vi "SS Current Test.vi"(6 "Lower Limit 2":dbl[](array[numeric])=[18.0, 18.0, 18.0, 18.0, 18.0, 18.0, 18.0, 18.0, 18.0, -1.0, -1.0, -1.0, -1.0, -1.0, -1.0, -1.0, -1.0, -1.0, 3.6, 3.6, 3.6, 3.6, 3.6, 3.6, -1.0, -1.0, -1.0, -1.0], 8 "Lower Limit":dbl[](array[numeric])=[18.0, 18.0, 18.0, 18.0, 18.0, 18.0, 18.0, 18.0, 18.0, -1.0, -1.0, -1.0, -1.0, -1.0, -1.0, -1.0, -1.0, -1.0, 3.6, 3.6, 3.6, 3.6, 3.6, 3.6, -1.0, -1.0, -1.0, -1.0], 9 "Y 2":dbl[](array[numeric]), 10 "Y":dbl[](array[numeric]), 11 "Upper Limit":dbl[](array[numeric])=[50.0, 50.0, 27.0, 27.0, 27.0, 27.0, 27.0, 27.0, 27.0, 27.0, 27.0, 1.0, 1.0, 1.0, 1.0, 1.0, 4.4, 4.4, 4.4, 4.4, 4.4, 4.4, 4.4, 4.4, 4.4, 4.4, 1.0, 1.0]) -> (2 "Out of Bounds":bool, 3 "Waveform Chart":waveform(dbl)[](graph))   [LabVIEW 2012]
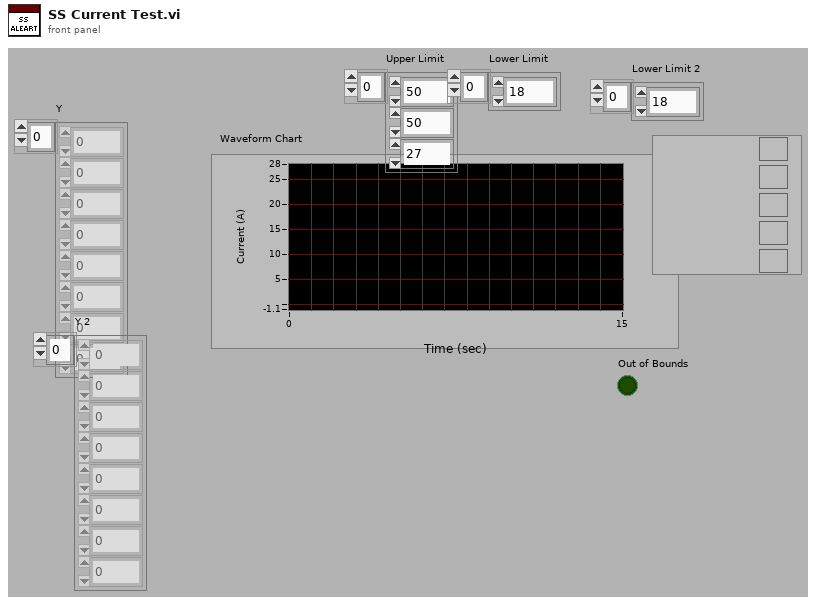
[diagram p1: front panel]
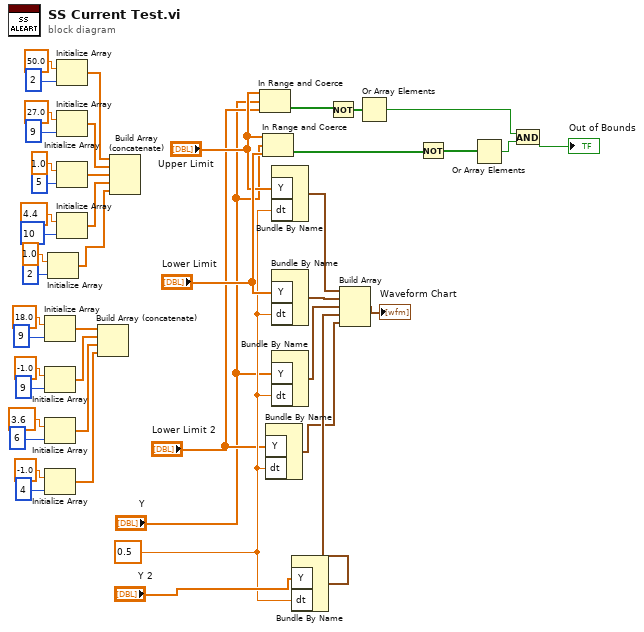
[diagram p0: block diagram]
diagram:
  w10 = 0.5 ("dt")
  n1 = Initialize Array(18.0, 9 ("dimension size")) -> (w30:dbl[])
  n2 = Initialize Array(-1.0, 9 ("dimension size")) -> (w29:dbl[])
  n3 = Initialize Array(3.6 ("y"), 6 ("dimension size")) -> (w28:dbl[])
  n4 = Initialize Array(-1.0, 4 ("dimension size")) -> (w27:dbl[])
  n5 = Initialize Array(1.0 ("y"), 2 ("dimension size")) -> (w13:dbl[])
  n6 = Initialize Array(50.0, 2 ("dimension size")) -> (w31:dbl[])
  n7 = Initialize Array(27.0, 9 ("dimension size")) -> (w32:dbl[])
  n8 = Initialize Array(1.0 ("y"), 5 ("dimension size")) -> (w33:dbl[])
  n9 = Initialize Array(4.4, 10 ("dimension size")) -> (w34:dbl[])
  n10 = Build Array (concatenate)(w30, w29, w28, w27) -> ()  [unwired: 1 out]
  n11 = Build Array (concatenate)(w31, w32, w33, w34, w13) -> ()  [unwired: 1 out]
  n12 = In Range and Coerce(upper limit="Upper Limit", x="Y", lower limit="Lower Limit 2") -> (In Range?=w5:bool[])  [unwired: 1 out]
  n13 = In Range and Coerce(upper limit="Upper Limit", x="Y", lower limit="Lower Limit") -> (In Range?=w17:bool[])  [unwired: 1 out]
  n14 = Bundle By Name("Y"="Lower Limit 2", "dt"=w10) -> (w9:waveform(dbl))  [unwired: 1 in]
  n15 = Bundle By Name("Y"="Upper Limit", "dt"=w10) -> (w46:waveform(dbl))  [unwired: 1 in]
  n16 = Bundle By Name("Y"="Lower Limit", "dt"=w10) -> (w44:waveform(dbl))  [unwired: 1 in]
  n17 = Bundle By Name("Y"="Y", "dt"=w10) -> (w43:waveform(dbl))  [unwired: 1 in]
  n18 = Bundle By Name("Y"="Y 2", "dt"=w10) -> (w11:waveform(dbl))  [unwired: 1 in]
  n19 = Not(x=w5) -> (.not. x?=w4:bool[])
  n20 = Build Array(w46, w44, w43, w11, w9) -> (→"Waveform Chart":waveform(dbl)[])
  n21 = Or Array Elements(Boolean array=w4) -> (logical OR=w1:bool)
  n22 = Not(x=w17) -> (.not. x?=w16:bool[])
  n23 = Or Array Elements(Boolean array=w16) -> (logical OR=w2:bool)
  n24 = And(x=w1, y=w2) -> (x .and. y?=→"Out of Bounds":bool)
